vi "FPGA_Latch_for_loop.vi"() -> ()   [LabVIEW 2020]
uses:
  <vilib>/rvi/interface/RandomDataEmulation/niFpgaRandomDataHandleErrors.vi
  <vilib>/rvi/DataTransferAndStorage/Container/XNode/niFpgaContainer.xnode
  <vilib>/rvi/interface/RandomDataEmulation/nirviRandomDataFpgaReadWriteTemplate.vi
  <vilib>/Platform/TimedLoop/XDataNode/wakeup.ctl
  <vilib>/Platform/TimedLoop/XDataNode/XDNodeRunTimeDep.lvlib
  <vilib>/Platform/TimedLoop/XDataNode/nitl_modes.ctl
  <vilib>/Platform/TimedLoop/XDataNode/timing_clust.ctl
  <vilib>/platform/TimedLoop/XDataNode/XDataNode.xnode
panel:
  out "Output Valid":bool
  out "sort time (us)":u32
  out "Timed Out? FIFO index":bool
  out "Timed Out? FIFO list":bool
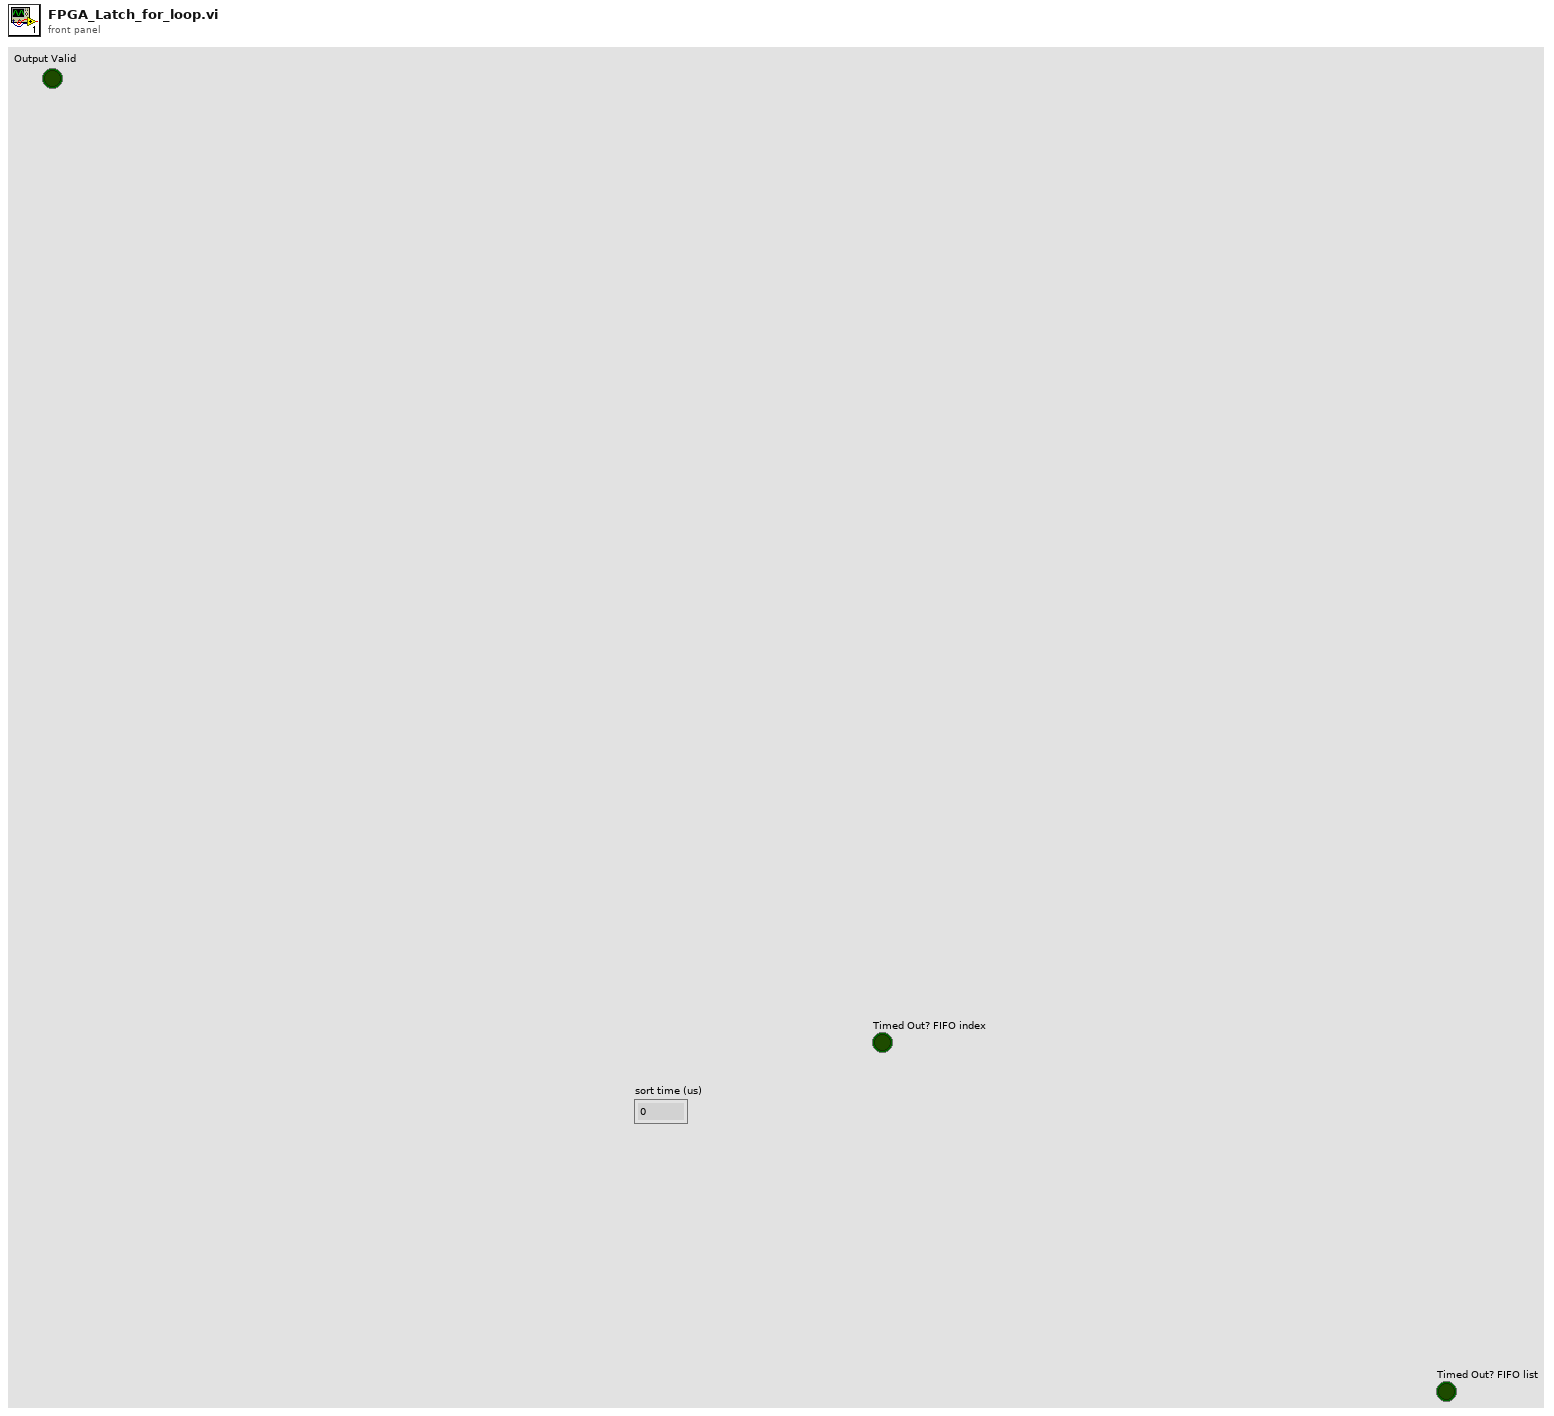
[diagram p1: front panel]
types:
  T1 = typedef "XDNodeRunTimeDep.lvlib/timing_clust.ctl" = cluster{"Expected End [f-1]":u64, "Actual End [f-1]":u64, "Finished Late? [f-1]":bool, "Expected End [i-1]":u64, "Actual End [i-1]":u64, "Finished Late? [i-1]":bool, "Expected Start [i]":u64, "Actual Start [i]":u64, "Expected Start [f]":u64, "Actual Start [f]":u64, "Source Name":string, "Structure Name":string, "Period":i64, "Deadline":i64, "Offset":i64, "Start":i64, "Priority":i32, "Timeout":i32, "Mode":T2, "Wakeup Reason":T3, "Error":errorcluster, "Source Type":string, "Secondary Source Type":string, "Global End Time":u64, "Global Start Time":u64, "Frame Duration":u64, "Iteration Duration":u64, "Assigned CPU":i32, "I/O Scan Engine Mode":u32}
  T2 = typedef "XDNodeRunTimeDep.lvlib/nitl_modes.ctl" = enum32{"No Change", "Process missed periods, maintain original phase", "Discard missed periods, maintain original phase", "Process missed periods, ignore original phase", "Discard missed periods, ignore original phase"}
  T3 = typedef "XDNodeRunTimeDep.lvlib/wakeup.ctl" = enum32{"Normal", "Aborted", "Asynchronous wakeup", "Timing source error", "Timed loop error", "Timeout"}
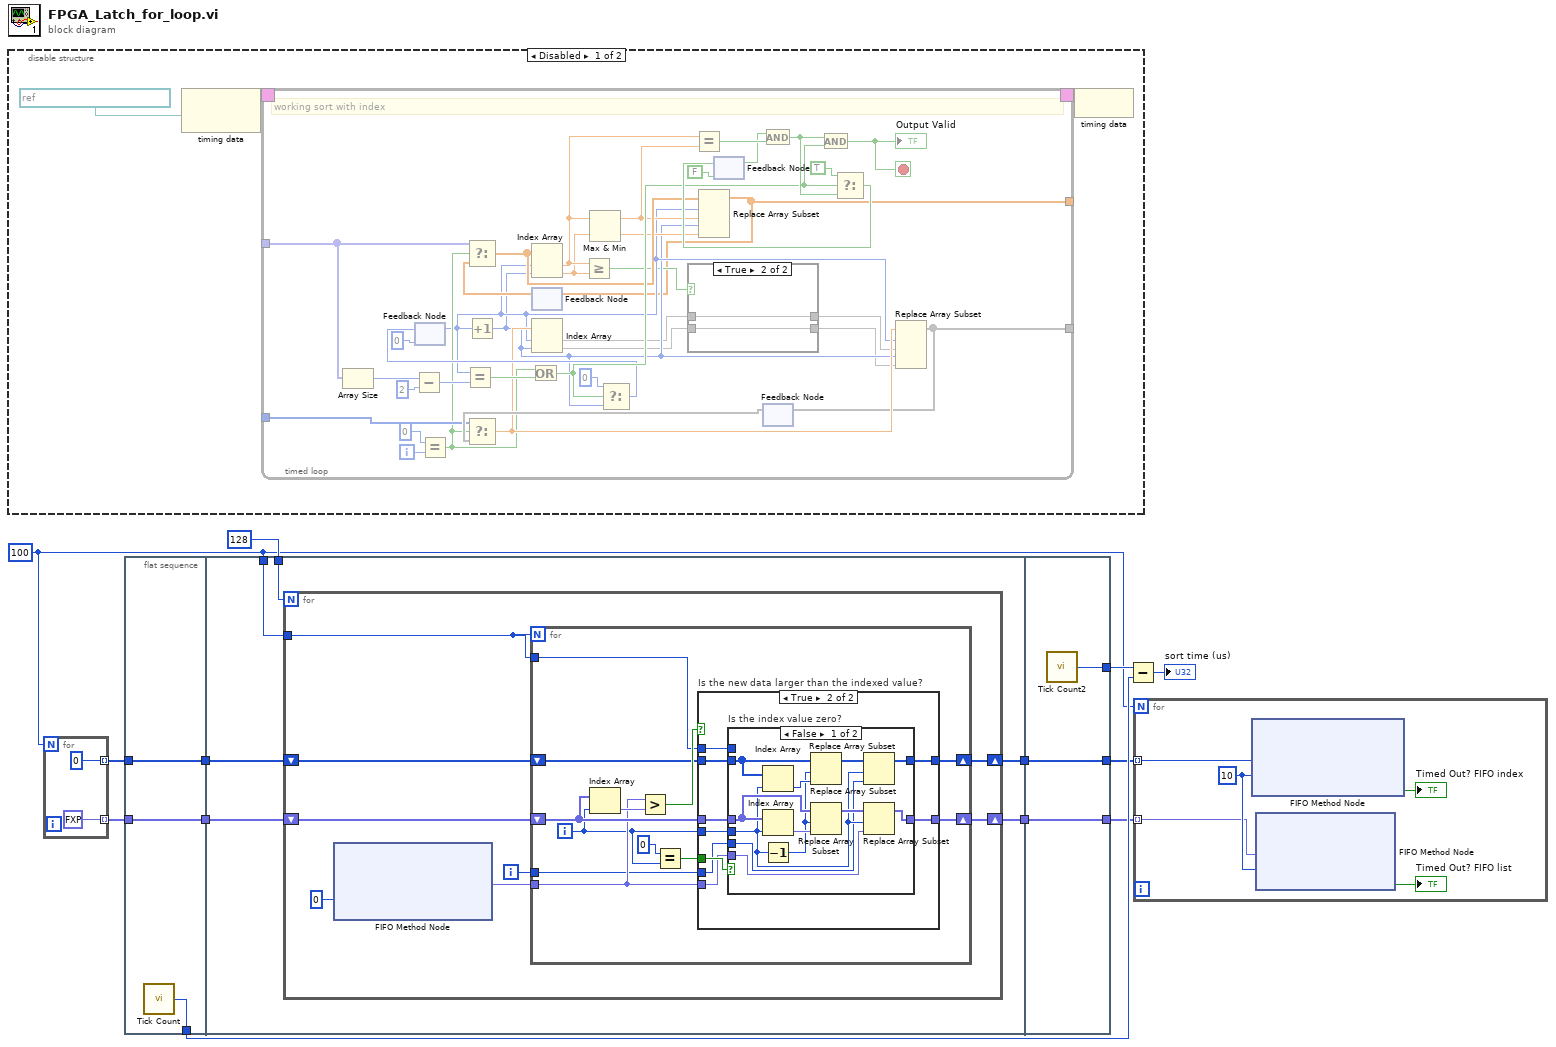
[diagram p0: block diagram]
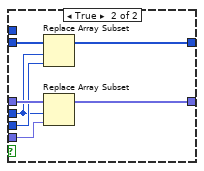
[diagram p5: hidden frame]
diagram:
  w1 = 100
  n1 = disable-structure shown="Disabled" {
    frame Disabled {
      n2 = node-c288(refnum<k21> "40 MHz Onboard Clock" ("Source Name")) -> (w17:T1)
      n3 = timed-loop {
        tunnel: _ -> [w51]
        tunnel: [w30] -> w15
        timing: w17 -> [_]
        timing-out: [_] -> w16
        tunnel: [w19] -> _
        tunnel: [w18] -> _
        i -> [w34]
        stop <- w35 stop-if-true
        # "working sort with index"
        n4 = Array Size(array=w51) -> (size(s)=w54:i32)
        n5 = Subtract(x=w54, y=2) -> (x-y=w52:i32)
        n6 = feedback #1(0 ("y")) -> (w28:i32)
        n7 = Equal?(x=0, y=w34) -> (x = y?=w29:bool)
        n8 = Equal?(x=w28, y=w52) -> (x = y?=w39:bool)
        n9 = Increment(x=w28) -> (x+1=w27:i32)
        n10 = Or(x=w29, y=w39) -> (x .or. y?=w42:bool)
        n11 = feedback #2() -> (w44:dbl[])  [unwired: 1 in]
        n12 = Select(t=w51, s=w29, f=w44) -> (s? t:f=w38:dbl[])
        n13 = Index Array(array=w38, index #1=w28, index #2=w27) -> (element #1=w22:dbl, element #2=w21:dbl)
        n14 = Greater Or Equal?(x=w22, y=w21) -> (x >= y?=w20:bool)
        n15 = Max & Min(x=w22, y=w21) -> (max(x,y)=w37:dbl, min(x,y)=w36:dbl)
        n16 = Select(t=0 ("y"), s=w42, f=w27) -> (s? t:f=w40:i32)
        n17 = feedback-in #1(w40) -> ()
        n18 = Equal?(x=w22, y=w37) -> (x = y?=w50:bool)
        n19 = Replace Array Subset(array=w38, new element #1=w37, index #1=w28, new element #2=w36, index #2=w27) -> (w19:dbl[])
        n20 = feedback-in #2(w19) -> ()
        n21 = feedback #3(FALSE ("t")) -> (w47:bool)
        n22 = And(x=w47, y=w50) -> (x .and. y?=w45:bool)
        n23 = feedback #4() -> (w32:void[])  [unwired: 1 in]
        n24 = Select(t=w30, s=w29, f=w32) -> (s? t:f=w31:dbl)
        n25 = Index Array(array=w31, index #1=w28, index #2=w27) -> (element #1=w26, element #2=w23)
        n26 = case shown="True" w20 {
          tunnel: w26 -> [w56 w58]
          tunnel: [w55 w58] -> w25
          tunnel: [w56 w57] -> w24
          tunnel: w23 -> [w55 w57]
          frame False {
          }
          frame True {
          }
        }
        n27 = And(x=w45, y=w42) -> (x .and. y?=w35:bool)
        "Output Valid" <- w35
        n28 = Select(t=TRUE, s=w42, f=w45) -> (s? t:f=w48:bool)
        n29 = feedback-in #3(w48) -> ()
        n30 = Replace Array Subset(array=w31, new element #1=w25, index #1=w28, new element #2=w24, index #2=w27) -> (w18:void[])
        n31 = feedback-in #4(w18) -> ()
      }
      n32 = node-c288(w16) -> ()
    }
    frame Enabled {
    }
  }
  n33 = for {
    N: w1 -> [_]
    tunnel: [fxp<+/-,32,21> 0.0 ("amplitude")] -> w7 mode=indexing
    tunnel: [0] -> w9 mode=indexing
  }
  n34 = flat-sequence {
    tunnel: [w69] -> w12
    tunnel: [w68] -> w10
    tunnel: w9 -> [w68]
    tunnel: [w67] -> w8
    tunnel: w7 -> [w67]
    tunnel: w10 -> [w75]
    tunnel: w8 -> [w74]
    tunnel: [w73] -> w6
    tunnel: [w72] -> w4
    tunnel: 128 ("samples") -> [w71]
    tunnel: w1 -> [w70]
    tunnel: [w128] -> w13
    tunnel: w6 -> [w127]
    tunnel: [w127] -> w5
    tunnel: w4 -> [w126]
    tunnel: [w126] -> w3
    frame #0 {
      n35 = call "Tick Count"() -> ("Tick Count(uSec)"=w69:u32)
    }
    frame #1 {
      n36 = for {
        N: w71 -> [_]
        shift-right: [w82] -> w73
        shift-left: w74 -> [w83]
        shift-right: [w80] -> w72
        shift-left: w75 -> [w79]
        tunnel: w70 -> [w76]
        i -> [w81]
        n37 = xnode ("FIFO Method Node")("Timeout"=0) -> ("Element"=w78:fxp<+/-,32,21>)  [unwired: 1 in, 2 out]
        n38 = for {
          N: w76 -> [_]
          tunnel: w78 -> [w92]
          tunnel: w76 -> [w90]
          shift-right: [w91] -> w82
          shift-left: w83 -> [w93]
          tunnel: w81 -> [w88]
          shift-right: [w86] -> w80
          shift-left: w79 -> [w87]
          i -> [w89]
          n39 = Index Array(array=w93, index=w89) -> (element=w95:fxp<+/-,32,21>)
          n40 = Greater?(x=w92, y=w95) -> (0:w94:bool)
          n41 = Equal?(x=0, y=w89) -> (x = y?=w84:bool)
          n42 = case "Is the new data larger than the indexed value?" shown="True" w94 {
            tunnel: w93 -> [w97 w105]
            tunnel: w84 -> [_ w106]
            tunnel: w90 -> [_ w104]
            tunnel: w92 -> [_ w103]
            tunnel: w89 -> [_ w102]
            tunnel: [w97 w101] -> w91
            tunnel: w88 -> [_ w100]
            tunnel: w87 -> [w96 w99]
            tunnel: [w96 w98] -> w86
            frame False {
            }
            frame True {
              n43 = case "Is the index value zero?" shown="False" w106 {
                tunnel: w105 -> [w118 w125]
                tunnel: w104 -> [_ _]
                tunnel: w103 -> [w115 w124]
                tunnel: w102 -> [w108 w121]
                tunnel: [w114 w123] -> w101
                tunnel: w100 -> [w107 w122]
                tunnel: w99 -> [w111 w120]
                tunnel: [w110 w119] -> w98
                frame False {
                  n44 = Index Array(array=w111, index=w108) -> (element=w113:i32)
                  n45 = Index Array(array=w118, index=w108) -> (element=w117:fxp<+/-,32,21>)
                  n46 = Decrement(x=w108) -> (x-1=w109:i32)
                  n47 = Replace Array Subset(array=w111, new element=w113, index=w109) -> (w112:i32[])
                  n48 = Replace Array Subset(array=w118, new element=w117, index=w109) -> (w116:fxp<+/-,32,21>[])
                  n49 = Replace Array Subset(array=w112, new element=w107, index=w108) -> (w110:i32[])
                  n50 = Replace Array Subset(array=w116, new element=w115, index=w108) -> (w114:fxp<+/-,32,21>[])
                }
                frame True {
                  n51 = Replace Array Subset(array=w120, new element=w122, index=w121) -> (w119:i32[])
                  n52 = Replace Array Subset(array=w125, new element=w124, index=w121) -> (w123:fxp<+/-,32,21>[])
                }
              }
            }
          }
        }
      }
    }
    frame #2 {
      n53 = call "Tick Count2"() -> ("Tick Count(uSec)"=w128:u32)
    }
  }
  n54 = Subtract(x=w13, y=w12) -> (x-y=→"sort time (us)":u32)
  n55 = for {
    N: w1 -> [_]
    tunnel: w5 -> [w130] mode=indexing
    tunnel: w3 -> [w129] mode=indexing
    w132 = 10 ("Timeout")
    n56 = xnode ("FIFO Method Node")("Element"=w129, "Timeout"=w132) -> ("Timed Out?"=→"Timed Out? FIFO index":bool)  [unwired: 1 in, 1 out]
    n57 = xnode ("FIFO Method Node")("Element"=w130, "Timeout"=w132) -> ("Timed Out?"=→"Timed Out? FIFO list":bool)  [unwired: 1 in, 1 out]
  }
